vi "SaveToFile.vi"(3 "Data":dbl[][](array[numeric]), 4 "Settings":T1={"Data Path"=path "", "Time"=timestamp(0 s since 1904-01-01), "Sampling Rate (Hz)"=44800, "Device"=0, "pre-trigger (sec)"=100.0, "length of sample (sec)"=1000.0, "trigger value (V)"=100.0, "Labels"=[], "Cutoffs (sec)"=[], "Freq Bands"=[]} {"Time" format="%<%H:%M\n%d/%m/%y>T"}, 5 "Path In":path) -> (2 "Path Out":path)   [LabVIEW 2014]
uses:
  <userlib>/CurtinCode/SettingsControl.ctl
panel:
  out "resulting string":string="Date: 03/12/31 19:00:00\nSampling rate(Hz): 44800\nDevice: 0\nCutoff (hammer): 100\nCutoff (microphones): 1000\nPoints before trigger: 100\nPoints after trigger: 1000\n\nHammer(V)\t microphone(V)\n-----------------------------\n"
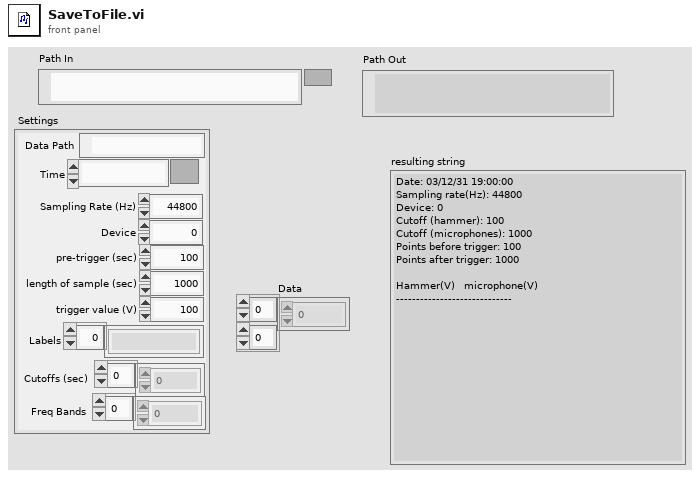
[diagram p1: front panel]
types:
  T1 = typedef "SettingsControl.ctl" = cluster{"Data Path":path, "Time":timestamp, "Sampling Rate (Hz)":u16, "Device":u16, "pre-trigger (sec)":dbl, "length of sample (sec)":dbl, "trigger value (V)":dbl, "Labels":string[], "Cutoffs (sec)":dbl[], "Freq Bands":dbl[]}
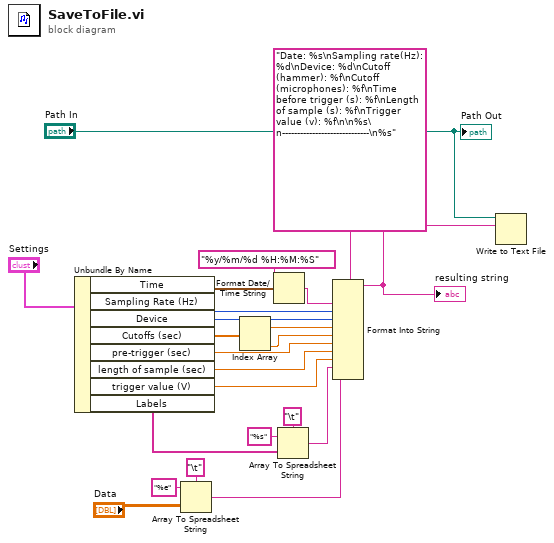
[diagram p0: block diagram]
diagram:
  n1 = Unbundle By Name("Settings") -> ("Time"=w18:timestamp, "Sampling Rate (Hz)"=w16:u16, "Device"=w15:u16, "Cutoffs (sec)"=w4:dbl[], "pre-trigger (sec)"=w14:dbl, "length of sample (sec)"=w13:dbl, "trigger value (V)"=w12:dbl, "Labels"=w8:string[])
  n2 = Array To Spreadsheet String(delimiter (Tab)="\t", array="Data", 3:"%e" ("format string")) -> (spreadsheet string=w9:string)
  n3 = Index Array(array=w4) -> (element #1=w3:dbl, element #2=w2:dbl)  [unwired: 2 in]
  n4 = Format Date/Time String(time format string (%c)="%y/%m/%d %H:%M:%S", seconds (now)=w18) -> (date/time string=w17:string)  [unwired: 1 in]
  n5 = Array To Spreadsheet String(delimiter (Tab)="\t", array=w8, 3:"%s" ("delimiter (Tab)")) -> (spreadsheet string=w7:string)
  n6 = Format Into String(format string="Date: %s\nSampling rate(Hz): %d\nDevice: %d\nCutoff (hammer): %f\nCutoff (microphones): %f\nTime before trigger (s): %f\nLength of sample (s): %f\nTrigger value (v): %f\n\n%s\n-----------------------------\n%s", w17, w16, w15, w3, w2, w14, w13, w12, w7, w9) -> (resulting string=w10:string)  [unwired: 2 in, 1 out]
  "resulting string" <- w10
  n7 = Write to Text File(file (use dialog)="Path In", text=w10) -> ()  [unwired: 2 in, 3 out]
  "Path Out" <- "Path In"
